vi "GuessTheNumber.vi"() -> ()   [LabVIEW 2018]
panel:
  in  "Guess":dbl
  in  "Max Number":dbl
  in  "Start Button":bool
  in  "stop":bool
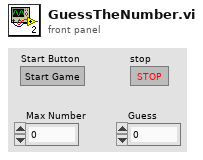
[diagram p1: front panel]
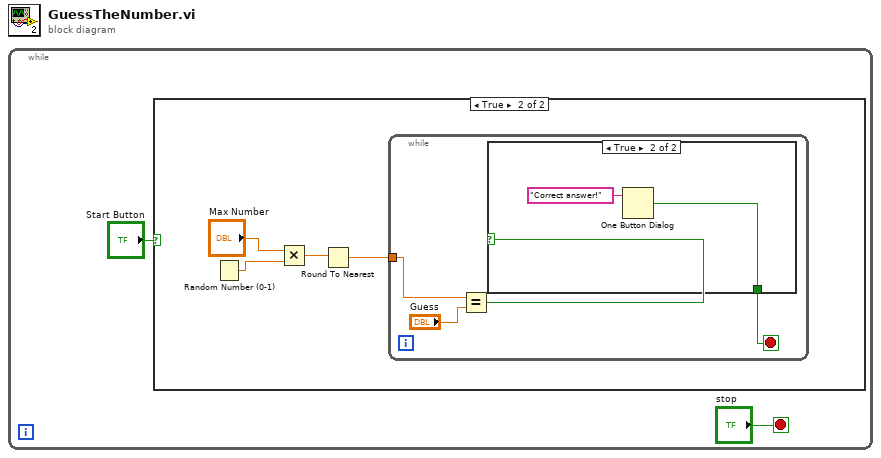
[diagram p0: block diagram]
diagram:
  n1 = while {
    stop <- "stop" stop-if-true
    n2 = case shown="True" "Start Button" {
      frame False {
      }
      frame True {
        n3 = Random Number (0-1)() -> (number: 0 to 1=w6:dbl)
        n4 = Multiply(x="Max Number", y=w6) -> (x*y=w4:dbl)
        n5 = Round To Nearest(number=w4) -> (nearest integer value=w3:dbl)
        n6 = while {
          tunnel: w3 -> [w10]
          stop <- w7 stop-if-true
          n7 = Equal?(x=w10, y="Guess") -> (x = y?=w8:bool)
          n8 = case shown="True" w8 {
            tunnel: [_ w11] -> w7
            frame False {
            }
            frame True {
              n9 = One Button Dialog(message="Correct answer!") -> (true=w11:bool)  [unwired: 1 in]
            }
          }
        }
      }
    }
  }
